vi "power_energy_param.vi"() -> ()   [LabVIEW 2018]
panel:
  in  "能量计量程":enum16{"200uJ", "20uJ", "2uJ", "200nJ"}(ring)
  in  "能量计通道":enum16{"Channel 1", "Channel 2"}(ring)=enum."Channel 2"
  in  "功率计通道":enum16{"Channel 1", "Channel 2"}(ring)
  in  "测量表头IP":string="192.168.129.77"
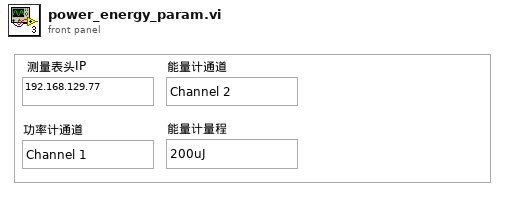
[diagram p1: front panel]
types:
  T1 = typedef "IMAQ Image.ctl" = refnum<image>
  T2 = cluster{"示波器":cluster{"Channel (0:Channel 1)":enum16{"Channel 1", "Channel 2", "Channel 3", "Channel 4"}, "电压范围":dbl, "触发电压":dbl, "时间范围":dbl, " 示波器VISA":refnum<visa-resource-name>}, "光谱仪":cluster{"Channel (0:Channel 1)":enum16{"Channel 1", "Channel 2", "Channel 3", "Channel 4"}, "电压范围":u64, "触发电压":u64, "时间范围":u64}, " 近场相机":cluster{"曝光时间":i32, "模拟增益":i32, "控制套接字":i32, "IP 地址":string, " 采集套接字":i32, "  版本号":i32, "ImageData":T1, "  增益最大":i32, "  增益最小":i32, " 曝光最大":i32, " 曝光最小":i32, " 帧速":i32, " 同步切换":i32, "  曝光缩放":i32}, " 偏振仪":cluster{"电压范围":u64, "触发电压":u64, "时间范围":u64, "波长范围":enum16{"可见光 400-700nm", "近红外 700-1100nm"}}, " 功率计":cluster{"通道":enum16{"Channel 1", "Channel 2"}, "工作波长":u32, "单位":u64, "时间范围":u64, "IP地址":string, "端口":u32}, "能量计":cluster{"通道":enum16{"Channel 1", "Channel 2"}, "工作波长":u32, "单位":u64, "时间范围":u64, "IP地址":string, "端口":u32, "能量计量程":enum16{"200uJ", "20uJ", "2uJ", "200nJ"}}, "电机":cluster{"Channel (0:Channel 1)":enum16{"Channel 1", "Channel 2", "Channel 3", "Channel 4"}, "电压范围":u64, "触发电压":u64, "时间范围":u64}}
  T3 = cluster{"通道":enum16{"Channel 1", "Channel 2"}, "工作波长":u32, "单位":u64, "时间范围":u64, "IP地址":string, "端口":u32}
  T4 = cluster{"通道":enum16{"Channel 1", "Channel 2"}, "工作波长":u32, "单位":u64, "时间范围":u64, "IP地址":string, "端口":u32, "能量计量程":enum16{"200uJ", "20uJ", "2uJ", "200nJ"}}
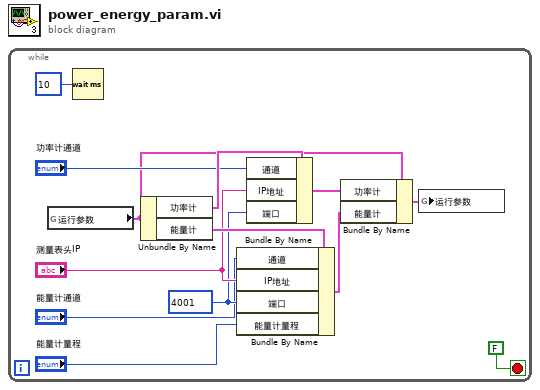
[diagram p0: block diagram]
diagram:
  n1 = while {
    stop <- FALSE stop-if-true
    w8 = u32 4001 ("端口")
    n2 = global read "参数.vi" "运行参数"() -> (w4:T2)
    n3 = Wait (ms)(milliseconds to wait=u32 10 ("等待时间（毫秒）")) -> ()  [unwired: 1 out]
    n4 = Unbundle By Name(w4) -> ("功率计"=w11:T3, "能量计"=w10:T4)
    n5 = Bundle By Name(cluster=w10, "通道"="能量计通道", "IP地址"="测量表头IP", "端口"=w8, "能量计量程"="能量计量程") -> (w3:T4)
    n6 = Bundle By Name(cluster=w11, "通道"="功率计通道", "IP地址"="测量表头IP", "端口"=w8) -> (w2:T3)
    n7 = Bundle By Name(cluster=w4, "功率计"=w2, "能量计"=w3) -> (w1:T2)
    n8 = global write "参数.vi" "运行参数"(w1) -> ()
  }
